vi "getType.vi"(8 "error in (no error)":errorcluster, 11 "Control in":refnum<class "Control.lvclass">) -> (0 "error out":errorcluster, 2 "type":refnum<vi>, 3 "Control out":refnum<class "Control.lvclass">)   [LabVIEW 2023, in "TLC_Scripto.lvlib" / "Control.lvclass"]
uses:
  Control.lvclass
  Control.lvclass/Control.ctl
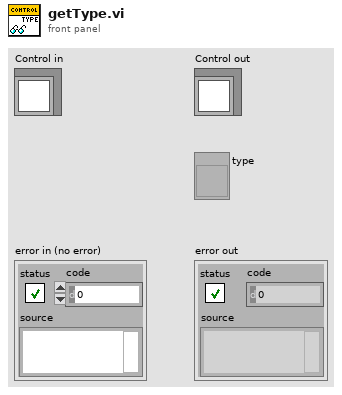
[diagram p1: front panel]
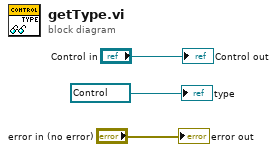
[diagram p0: block diagram]
diagram:
  "error out" <- "error in (no error)"
  "Control out" <- "Control in"
  "type" <- refnum<vi> refnum ("type")
